vi "PDE Thermal Distribution_Gen Boundary Plot.vi"(8 "Y":T2={"start y"=0.0, "end y"=1.0, "# of y-points"=11}, 9 "X":T3={"start x"=0.0, "end x"=1.0, "# of x-points"=11}, 10 "index (time step)":i32=-1, 11 "U(t, x, y)":dbl[][][](array[numeric])) -> (0 "End Y":T1(graph), 1 "Start Y":T1(graph), 2 "End X":T1(graph), 3 "Start X":T1(graph))   [LabVIEW 2023]
doc: "Generate boundary plot for PDE Thermal Distribution.vi example."
uses:
  <vilib>/Analysis/1siggen.llb/Ramp Pattern by Samples.vi
  <vilib>/gmath/NI_PDE.lvlib
  <vilib>/Analysis/NI_AALBase.lvlib
panel:
  out "Solution":dbl[][](graph)
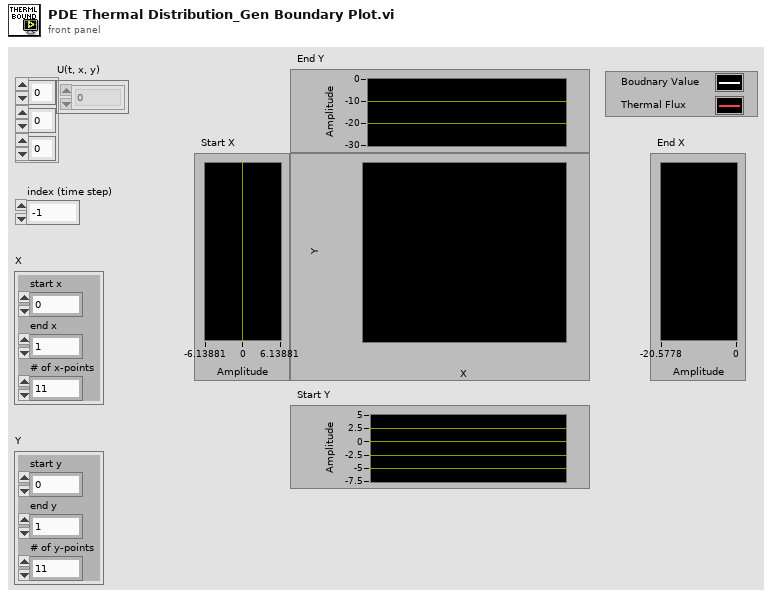
[diagram p1: front panel]
types:
  T1 = cluster{"Ramp Pattern":dbl[], "U(t, x, y)":dbl[]}[]
  T2 = cluster{"start y":dbl, "end y":dbl, "# of y-points":i32}
  T3 = cluster{"start x":dbl, "end x":dbl, "# of x-points":i32}
  T4 = cluster{"Ramp Pattern":dbl[], "U(t, x, y)":dbl[]}
  T5 = cluster{"U(t, x, y)":dbl[], "Ramp Pattern":dbl[]}
  T6 = cluster{"U(t, x, y)":dbl[], "Ramp Pattern":dbl[]}[]
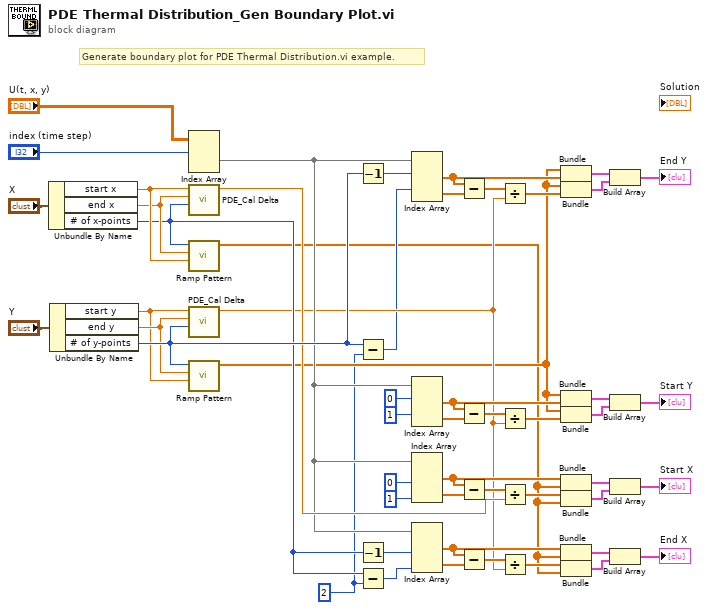
[diagram p0: block diagram]
diagram:
  w1 = 2 ("y")
  # "Generate boundary plot for PDE Thermal Distribution.vi example."
  n1 = Unbundle By Name("X") -> ("start x"=w45:dbl, "end x"=w44:dbl, "# of x-points"=w14:i32)
  n2 = Unbundle By Name("Y") -> ("start y"=w47:dbl, "end y"=w48:dbl, "# of y-points"=w49:i32)
  n3 = Index Array(array="U(t, x, y)", index (dim 0)="index (time step)") -> (element=w15:dbl[][])  [unwired: 2 in]
  n4 = call <vilib>:"PDE_Cal Delta.vi"("# of points"=w14, "end"=w44, "start"=w45) -> ("delta"=w25:dbl)  [unwired: 8 out]
  n5 = call-poly <vilib>:"Ramp Pattern.vi"("start"=w45, "end"=w44, "samples"=w14) -> ("Ramp Pattern"=w2:dbl[])  [unwired: 7 in, 1 out]
  n6 = call <vilib>:"PDE_Cal Delta.vi"("# of points"=w49, "end"=w48, "start"=w47) -> ("delta"=w13:dbl)  [unwired: 8 out]
  n7 = call-poly <vilib>:"Ramp Pattern.vi"("start"=w47, "end"=w48, "samples"=w49) -> ("Ramp Pattern"=w3:dbl[])  [unwired: 7 in, 1 out]
  n8 = Decrement(x=w49) -> (x-1=w10:i32)
  n9 = Subtract(x=w49, y=w1) -> (x-y=w11:i32)
  n10 = Decrement(x=w14) -> (x-1=w20:i32)
  n11 = Subtract(x=w14, y=w1) -> (x-y=w21:i32)
  n12 = Index Array(array=w15, index (row) #1=w10, index (row) #2=w11) -> (element #1=w7:dbl[], element #2=w9:dbl[])  [unwired: 2 in]
  n13 = Index Array(array=w15, index (row) #1=0 ("y"), index (row) #2=1 ("y")) -> (element #1=w37:dbl[], element #2=w35:dbl[])  [unwired: 2 in]
  n14 = Index Array(array=w15, index (col) #1=0 ("y"), index (col) #2=1 ("y")) -> (element #1=w32:dbl[], element #2=w26:dbl[])  [unwired: 2 in]
  n15 = Index Array(array=w15, index (col) #1=w20, index (col) #2=w21) -> (element #1=w23:dbl[], element #2=w16:dbl[])  [unwired: 2 in]
  n16 = Subtract(x=w7, y=w9) -> (x-y=w8:dbl[])
  n17 = Subtract(x=w37, y=w35) -> (x-y=w36:dbl[])
  n18 = Subtract(x=w32, y=w26) -> (x-y=w27:dbl[])
  n19 = Subtract(x=w23, y=w16) -> (x-y=w17:dbl[])
  n20 = Divide(x=w8, y=w13) -> (x/y=w6:dbl[])
  n21 = Divide(x=w36, y=w13) -> (x/y=w38:dbl[])
  n22 = Divide(x=w27, y=w25) -> (x/y=w33:dbl[])
  n23 = Divide(x=w17, y=w13) -> (x/y=w22:dbl[])
  n24 = Bundle("Ramp Pattern"=w3, "U(t, x, y)"=w7) -> (w5:T4)  [unwired: 1 out]
  n25 = Bundle("Ramp Pattern"=w3, w6) -> (w4:cluster{"Ramp Pattern":dbl[], dbl[]})  [unwired: 1 out]
  n26 = Bundle("Ramp Pattern"=w3, "U(t, x, y)"=w37) -> (w39:T4)  [unwired: 1 out]
  n27 = Bundle("Ramp Pattern"=w3, w38) -> (w40:cluster{"Ramp Pattern":dbl[], dbl[]})  [unwired: 1 out]
  n28 = Bundle("U(t, x, y)"=w32, "Ramp Pattern"=w2) -> (w28:T5)  [unwired: 1 out]
  n29 = Bundle(w33, "Ramp Pattern"=w2) -> (w29:cluster{dbl[], "Ramp Pattern":dbl[]})  [unwired: 1 out]
  n30 = Bundle("U(t, x, y)"=w23, "Ramp Pattern"=w2) -> (w18:T5)  [unwired: 1 out]
  n31 = Bundle(w22, "Ramp Pattern"=w2) -> (w19:cluster{dbl[], "Ramp Pattern":dbl[]})  [unwired: 1 out]
  n32 = Build Array(w5, w4) -> (→"End Y":T1)
  n33 = Build Array(w39, w40) -> (→"Start Y":T1)
  n34 = Build Array(w28, w29) -> (→"Start X":T6)
  n35 = Build Array(w18, w19) -> (→"End X":T6)
